vi "Read MusicLibrary.vi"(8 "error in (no error)":errorcluster, 11 "MusicFile in":refnum<class "MusicFile.lvclass">) -> (0 "error out":errorcluster, 2 "MusicLibrary.lvclass":refnum<class "MusicLibrary.lvclass">, 3 "MusicFile out":refnum<class "MusicFile.lvclass">)   [LabVIEW 2015, in "MusicFile.lvclass"]
uses:
  MusicFile.lvclass
  MusicElementLibrary/MusicLibrary/MusicLibrary.lvclass
  MusicFile.lvclass/MusicFile.ctl
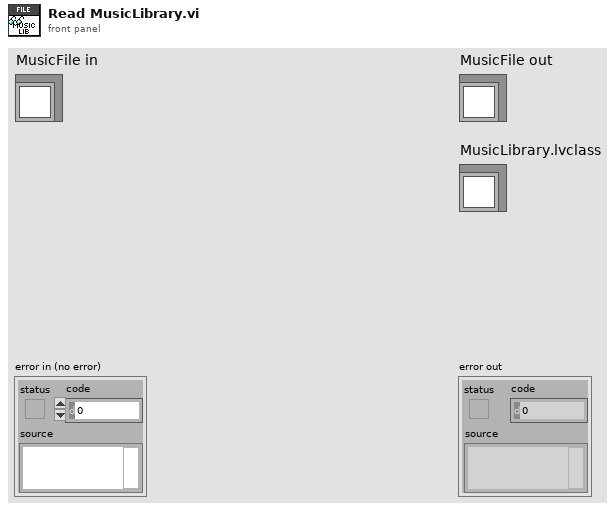
[diagram p1: front panel]
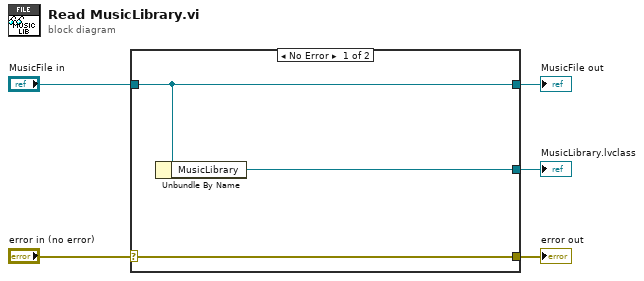
[diagram p0: block diagram]
diagram:
  n1 = case shown="No Error" "error in (no error)" {
    selector: "error in (no error)" -> [w8 w9]
    tunnel: [w8 w9] -> w4
    tunnel: [w7 w10] -> w2
    tunnel: "MusicFile in" -> [w7 w10]
    tunnel: [w6 _] -> w1
    frame No Error {
      n2 = Unbundle By Name(w7) -> ("MusicLibrary"=w6:refnum<class "MusicLibrary.lvclass">)
    }
    frame Error {
    }
  }
  "error out" <- w4
  "MusicFile out" <- w2
  "MusicLibrary.lvclass" <- w1
